vi "OptionCycle.vi"(8 "MinValue":i32, 9 "MaxValue":i32, 10 "BackwardsInput":bool, 11 "ForwardInput":bool) -> (3 "CycleNum":i32)   [LabVIEW 2020]
doc: "Cycles through a series of integer values based on a boolean input to either incremet or decrement the value. To obtain a single cycle input, recommend using \"EdgeOn.vi\" to detect whena button is pressed. \n\nInputs:\n-- ForwardInput -- Boolean -- Send a true value to increment the series by 1 --\n-- BackwardsInput -- Boolean -- Send a true value to decrement the series by 1 --\n-- MaxValue -- Integer -- The maximum value of the series (Inclusive) --\n-- MinValue -- Double -- The minimum value of the series (Exclusive) --\n\nOutputs:\n-- CycleNum -- Integer -- The current location in the series --"
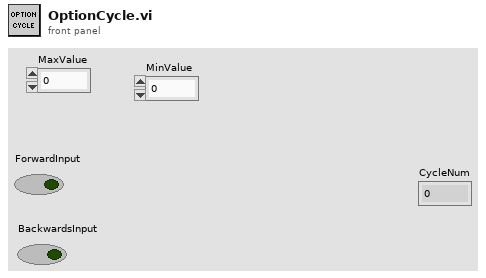
[diagram p1: front panel]
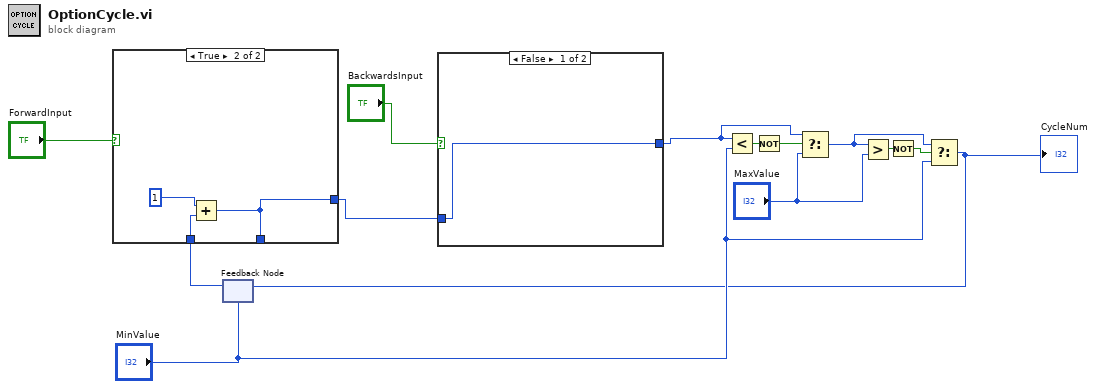
[diagram p0: block diagram]
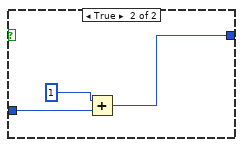
[diagram p2: hidden frame]
diagram:
  n1 = feedback #1("MinValue") -> (w12:i32)
  n2 = case shown="True" "ForwardInput" {
    tunnel: [w14 w15] -> _
    tunnel: w12 -> [w14 w16]
    tunnel: [w14 w15] -> w10
    frame False {
    }
    frame True {
      n3 = Add(x=1, y=w16) -> (x+y=w15:i32)
    }
  }
  n4 = case shown="False" "BackwardsInput" {
    tunnel: [w18 w20] -> w7
    tunnel: w10 -> [w18 w19]
    frame False {
    }
    frame True {
      n5 = Add(x=1, y=w19) -> (x+y=w20:i32)
    }
  }
  n6 = Less?(x=w7, y="MinValue") -> (x < y?=w9:bool)
  n7 = Not(x=w9) -> (.not. x?=w8:bool)
  n8 = Select(t=w7, s=w8, f="MaxValue") -> (s? t:f=w4:i32)
  n9 = Greater?(x=w4, y="MaxValue") -> (0:w6:bool)
  n10 = Not(x=w6) -> (.not. x?=w5:bool)
  n11 = Select(t=w4, s=w5, f="MinValue") -> (s? t:f=w1:i32)
  "CycleNum" <- w1
  n12 = feedback-in #1(w1) -> ()
